vi "A180648.vi"() -> ()   [LabVIEW 2020]
panel:
  in  "磨合曲线":refnum<vi>
  in  "LED-磨合":refnum<vi>
  in  "磨合参数":string[][](table)=[[""], ["°/S"], ["°"], ["Nm"]]
  in  "逆向空载参数":string[][](table)=[[""], ["°/S"], ["°"], ["Nm"]]
  in  "磨合试验参数":T1
  out "力特性参数":sgl[](array[numeric])
  out "当前车速":u16
  out "车速":sgl[](array[numeric])
  in  "振动NVH-FFT曲线":refnum<vi>
  in  "工位二复检曲线":refnum<vi>
  in  "工位一复检曲线":refnum<vi>
  in  "CAN_CYCLE":T2(array[cluster]) {"周期(ms)" min=1 format="%d ms"; "ID" format="0x%x"}
  in  "功能试验参数":T3
  in  "逆向空载试验参数":T1
  in  "当前检测项":enum32{"拉轴", "卡簧", "完成"}(ring)
  out "检测结果":string[][][](array[string])
  in  "力特性":T4
  in  "空载":T5
  in  "逆向空载曲线":refnum<vi>
  in  "振动NVH-Order曲线":refnum<vi>
  in  "电流特性曲线":refnum<vi>
  in  "LED-逆向空载":refnum<vi>
  in  "LED-振动NVH":refnum<vi>
  in  "LED-电流特性":refnum<vi>
  in  "功能":T6
  in  "侧铆曲线":refnum<vi>
  in  "LED-传感器特性":refnum<vi>
  in  "LED-端铆":refnum<vi>
  in  "LED-侧铆":refnum<vi>
  in  "LED-轴承压装":refnum<vi>
  in  "试验项":T7(tab)
  in  "压装曲线":refnum<vi>
  in  "45°曲线":refnum<vi>
  in  "0°曲线":refnum<vi>
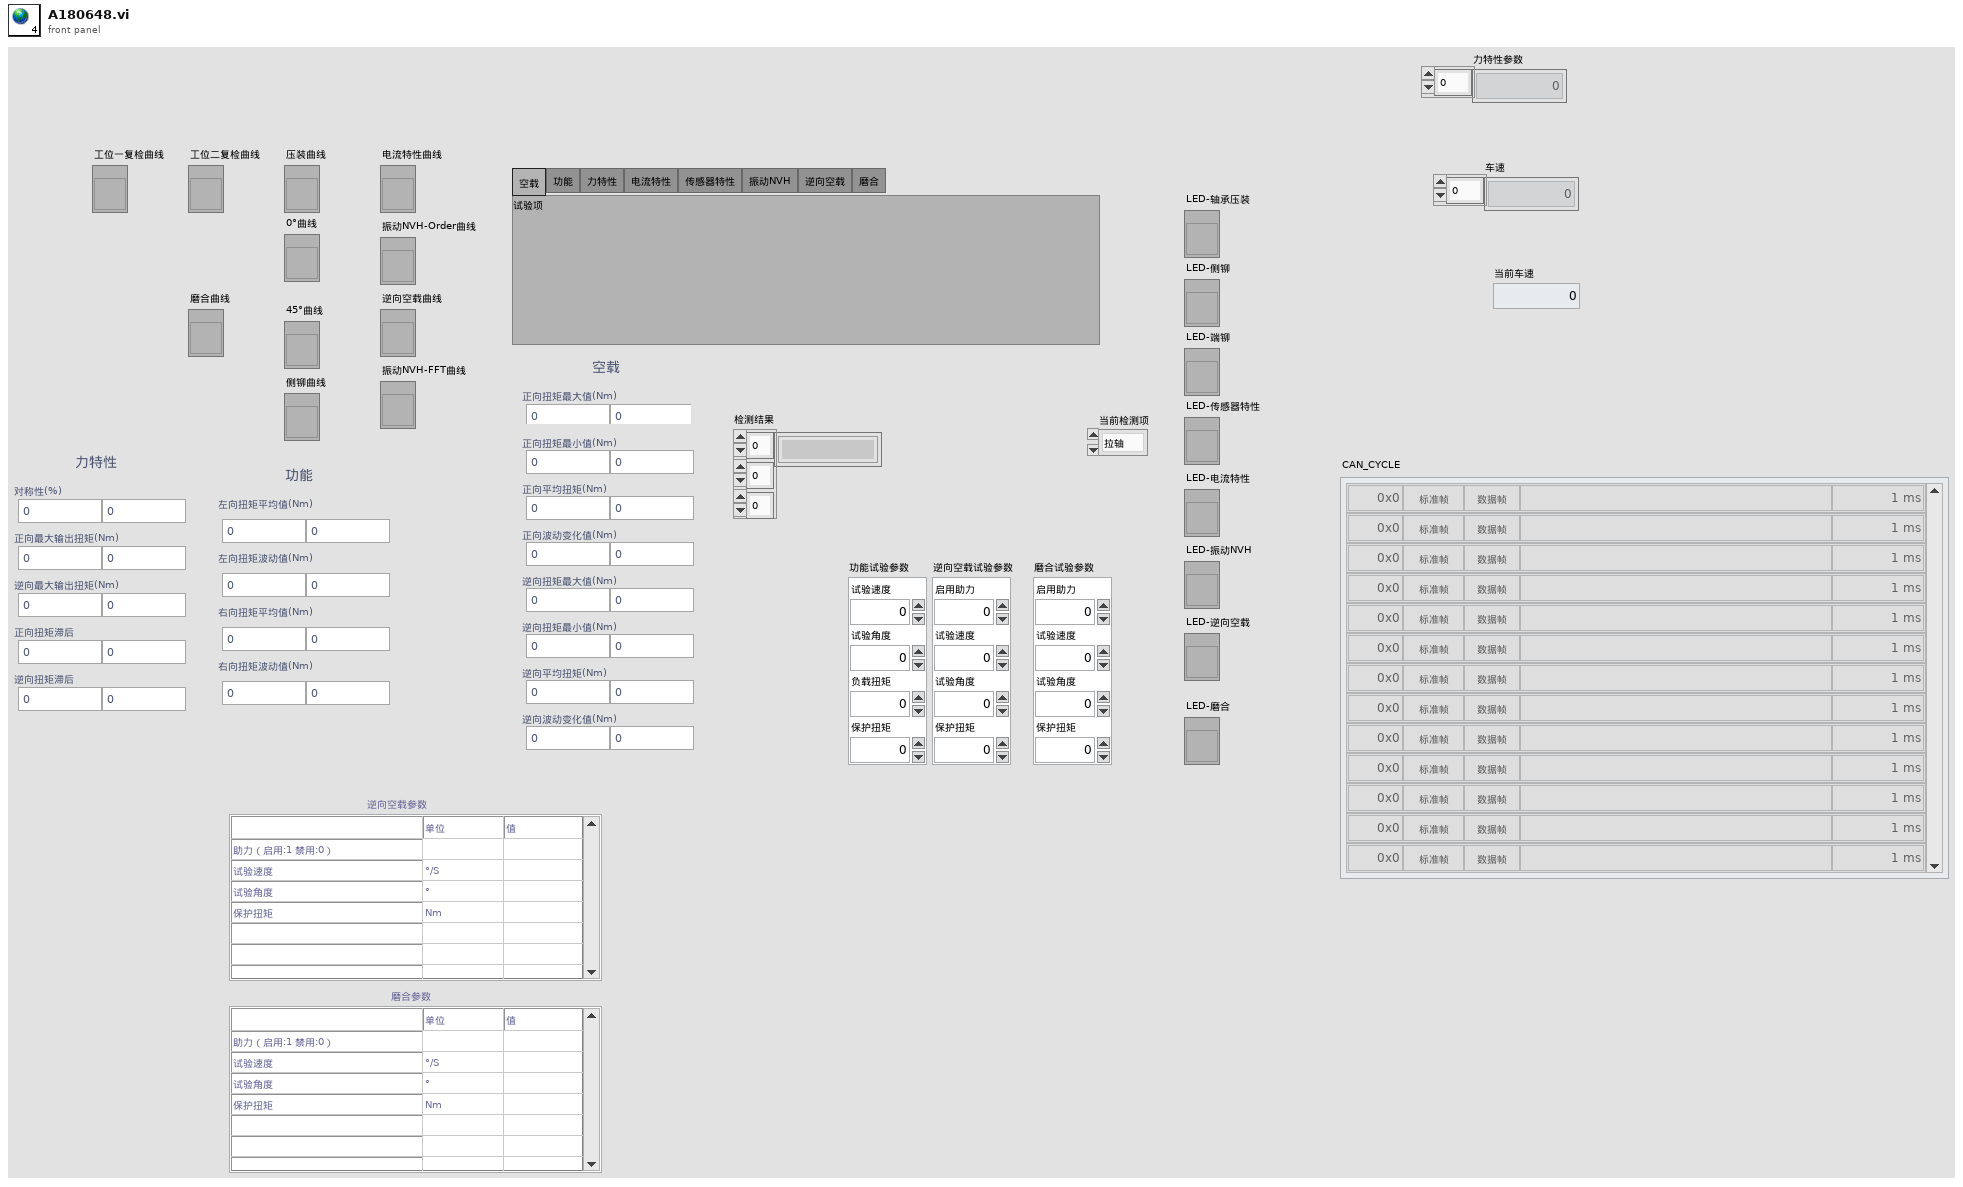
[diagram p1: front panel]
types:
  T1 = cluster{"启用助力":dbl, "试验速度":dbl, "试验角度":dbl, "保护扭矩":dbl}
  T2 = cluster{"ID":u32, "帧类型":enum8{"标准帧", "扩展帧"}, "帧格式":enum16{"数据帧", "远程帧"}, "帧数据":string, "周期(ms)":u32}[]
  T3 = cluster{"试验速度":dbl, "试验角度":dbl, "负载扭矩":dbl, "保护扭矩":dbl}
  T4 = cluster{"对称性(%)":cluster{"下限":dbl, "上限":dbl}, "正向最大输出扭矩(Nm)":cluster{"下限":dbl, "上限":dbl}, "逆向最大输出扭矩(Nm)":cluster{"下限":dbl, "上限":dbl}, "正向扭矩滞后":cluster{"下限":dbl, "上限":dbl}, "逆向扭矩滞后":cluster{"下限":dbl, "上限":dbl}}
  T5 = cluster{"正向扭矩最大值(Nm)":cluster{"下限":dbl, "上限":dbl}, "正向扭矩最小值(Nm)":cluster{"下限":dbl, "上限":dbl}, "正向平均扭矩(Nm)":cluster{"下限":dbl, "上限":dbl}, "正向波动变化值(Nm)":cluster{"下限":dbl, "上限":dbl}, "逆向扭矩最大值(Nm)":cluster{"下限":dbl, "上限":dbl}, "逆向扭矩最小值(Nm)":cluster{"下限":dbl, "上限":dbl}, "逆向平均扭矩(Nm)":cluster{"下限":dbl, "上限":dbl}, "逆向波动变化值(Nm)":cluster{"下限":dbl, "上限":dbl}}
  T6 = cluster{"左向扭矩平均值(Nm)":cluster{"下限":dbl, "上限":dbl}, "左向扭矩波动值(Nm)":cluster{"下限":dbl, "上限":dbl}, "右向扭矩平均值(Nm)":cluster{"下限":dbl, "上限":dbl}, "右向扭矩波动值(Nm)":cluster{"下限":dbl, "上限":dbl}}
  T7 = enum32{"空载", "功能", "力特性", "电流特性", "传感器特性", "振动NVH", "逆向空载", "磨合"}
diagram:
